vi "Double to RGB Image.vi"(8 "error in (no error)":errorcluster, 9 "minimum":dbl, 10 "maximum":dbl, 11 "Image Reference In":T1) -> (0 "error out":errorcluster, 3 "Image Reference Out":T1)   [LabVIEW 2016]
doc: "This VI converts a double image to a U8 image by converting the pixels from values in a particular range to 0-255 and adding them to a new image."
uses:
  <vilib>/vision/Image Controls.llb/IMAQ Image.ctl
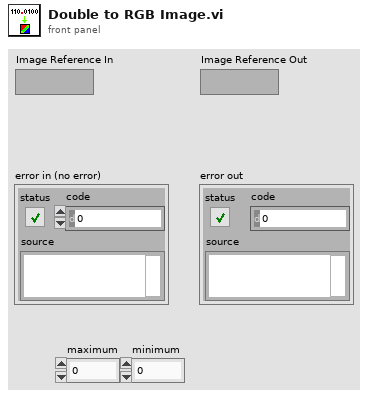
[diagram p1: front panel]
types:
  T1 = typedef "IMAQ Image.ctl" = refnum<image>
  T2 = typedef "Image Type" = u32
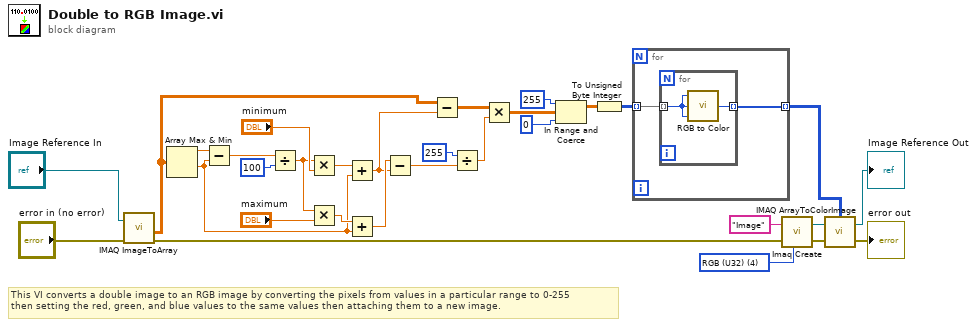
[diagram p0: block diagram]
diagram:
  w23 = T2 4 items=["Grayscale (U8)", "Grayscale (I16)", "Grayscale (SGL)", "Complex (CSG)", "RGB (U32)", "HSL (U32)", "RGB (U64)", "Grayscale (U16)"] ("Image Type")
  # "This VI converts a double image to an RGB image by converting the pixels from values in a particular range to 0-255\nthen setting the red, green, and blue values to the same values then attaching them to a new image."
  n1 = call "IMAQ ImageToArray"("error in (no error)"="error in (no error)", "Image"="Image Reference In") -> ("Image Pixels (Float)"=w27:sgl[][], "error out"=w18:errorcluster)  [unwired: 2 in, 3 out]
  n2 = Array Max & Min(array=w27) -> (max value=w28:sgl, min value=w5:sgl)  [unwired: 2 out]
  n3 = Subtract(x=w28, y=w5) -> (x-y=w14:sgl)
  n4 = Divide(x=w14, y=100) -> (x/y=w11:sgl)
  n5 = Multiply(x=w11, y="minimum") -> (x*y=w10:dbl)
  n6 = Multiply(x=w11, y="maximum") -> (x*y=w9:dbl)
  n7 = Add(x=w10, y=w5) -> (x+y=w6:dbl)
  n8 = Add(x=w9, y=w5) -> (x+y=w8:dbl)
  n9 = Subtract(x=w8, y=w6) -> (x-y=w7:dbl)
  n10 = Subtract(x=w27, y=w6) -> (x-y=w29:dbl[][])
  n11 = Divide(x=255, y=w7) -> (x/y=w31:dbl)
  n12 = Multiply(x=w29, y=w31) -> (x*y=w2:dbl[][])
  n13 = In Range and Coerce(upper limit=255, x=w2, lower limit=0) -> (coerced(x)=w1:dbl[][])  [unwired: 1 out]
  n14 = To Unsigned Byte Integer(number=w1) -> (unsigned 8bit integer=w22:u8[][])
  n15 = for {
    tunnel: w22 -> [w33] mode=indexing
    tunnel: [w32] -> w21 mode=indexing
    n16 = for {
      tunnel: w33 -> [w35] mode=indexing
      tunnel: [w34] -> w32 mode=indexing
      n17 = call <vilib>:"RGB to Color.vi"("B"=w35, "G"=w35, "R"=w35) -> ("Color"=w34:u32)
    }
  }
  n18 = call "Imaq Create"("Image Name"="Image", "Image Type"=w23, "error in (no error)"=w18) -> ("New Image"=w20:T1, "error out"=w19:errorcluster)  [unwired: 2 in]
  n19 = call "IMAQ ArrayToColorImage"("Image Pixels (U32)"=w21, "Image"=w20, "error in (no error)"=w19) -> ("Image Out"=→"Image Reference Out":T1, "error out"=→"error out":errorcluster)  [unwired: 2 in]
